vi "Symmetrical Components.vi"(8 "error in (no error)":errorcluster, 11 "3-phase phasors":cdb[](array[numeric])) -> (0 "error out":errorcluster, 1 "negative sequence":cdb, 2 "positive sequence":cdb, 3 "zero sequence":cdb)   [LabVIEW 2013, in "NI_EP_Basic.lvlib"]
doc: "Calculates the zero, positive, and negative sequence components of a three-phase electrical power system."
uses:
  <vilib>/addons/Electrical Power/Basic/NI_EP_Basic.lvlib
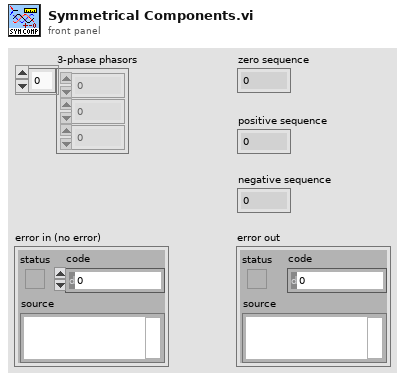
[diagram p1: front panel]
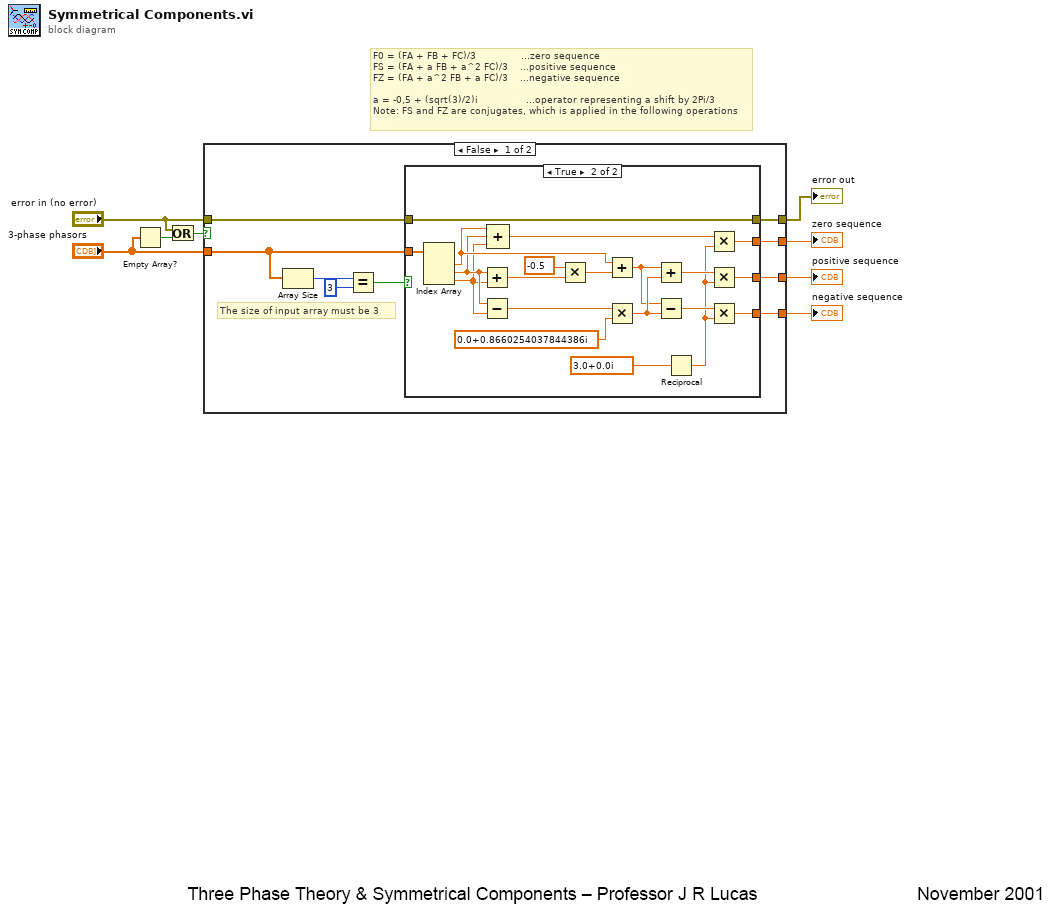
[diagram p0: block diagram]
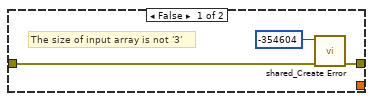
[diagram p2: hidden frame]
diagram:
  # "F0 = (FA + FB + FC)/3               ...zero sequence\nFS = (FA + a FB + a^2 FC)/3    ...positive sequence\nFZ = (FA + a^2 FB + a FC)/3    ...negative sequence\n\na = -0,5 + (sqrt(3)/2)i                ...operator representing a shift by 2Pi/3\nNote: FS and FZ are conjugates, which is applied in the following operations"
  n1 = Empty Array?(array="3-phase phasors") -> (empty?=w2:bool)
  n2 = Or(x="error in (no error)", y=w2) -> (x .or. y?=w4:bool)
  n3 = case shown="False" w4 {
    tunnel: "3-phase phasors" -> [w12 _]
    tunnel: [w17 _] -> w8
    tunnel: [w16 _] -> w7
    tunnel: [w15 _] -> w6
    tunnel: [w10 w41] -> w5
    tunnel: "error in (no error)" -> [w9 w41]
    frame False {
      # "The size of input array must be 3"
      n4 = Array Size(array=w12) -> (size(s)=w13:i32)
      n5 = Equal?(x=w13, y=3) -> (x = y?=w11:bool)
      n6 = case shown="True" w11 {
        tunnel: [_ w24] -> w17
        tunnel: [_ w23] -> w16
        tunnel: [_ w22] -> w15
        tunnel: w12 -> [_ w25]
        tunnel: [w19 w21] -> w10
        tunnel: w9 -> [w20 w21]
        frame False {
          # "The size of input array is not '3'"
          n7 = call <vilib>:"shared_Create Error.vi"("error in (no error)"=w20, "error code (0)"=-354604) -> ("error out"=w19:errorcluster)  [unwired: 9 in]
        }
        frame True {
          n8 = Index Array(array=w25) -> (element #1=w28:cdb, element #2=w27:cdb, element #3=w26:cdb)  [unwired: 3 in]
          n9 = Add(x=w27, y=w26) -> (x+y=w32:cdb)
          n10 = Subtract(x=w27, y=w26) -> (x-y=w35:cdb)
          n11 = Compound Arithmetic op=ADD(w28, w27, w26) -> (w30:cdb)
          n12 = Multiply(x=-0.5 ("y"), y=w32) -> (x*y=w34:cdb)
          n13 = Add(x=w28, y=w34) -> (x+y=w37:cdb)
          n14 = Multiply(x=w35, y=cdb 0.0+0.8660254037844386i) -> (x*y=w38:cdb)
          n15 = Add(x=w37, y=w38) -> (x+y=w39:cdb)
          n16 = Subtract(x=w37, y=w38) -> (x-y=w40:cdb)
          n17 = Reciprocal(x=cdb 3.0+0.0i ("y")) -> (1/x=w31:cdb)
          n18 = Multiply(x=w30, y=w31) -> (x*y=w22:cdb)
          n19 = Multiply(x=w39, y=w31) -> (x*y=w24:cdb)
          n20 = Multiply(x=w40, y=w31) -> (x*y=w23:cdb)
        }
      }
    }
    frame True {
    }
  }
  "positive sequence" <- w8
  "negative sequence" <- w7
  "zero sequence" <- w6
  "error out" <- w5
